vi "BRA_Query.vi"(0 "System no.":i32=1 min=1 max=4 step=1, 2 "Axes to query":string[](array[string]), 3 "Invert order?":bool, 4 "Query status of all brakes?":bool, 5 "error in":errorcluster) -> (14 "Axes with brake":string[](array[string]), 15 "Brake status?":bool[](array[boolean]), 19 "error out":errorcluster)   [LabVIEW 2020]
doc: "Returns list of axes with a brake and status of the brakes for queried axes. Requires SPA?.vi to be present.\n\nC-843, C-843.PM, C-844, Mercury: Invert order should be FALSE. Brake status? is not valid.\n\nC-848, C-880: Invert order should be TRUE. Brake status? is not valid\n\nC-884, C-891, Mercury_GCS: Invert order is not valid. VI returns axes with brakes and their brake status."
uses:
  Global1.vi
  Global2 (Array).vi
panel:
  # "Returns list of axes with a brake and status of the brakes for queried axes.  Requires \nSPA?.vi to be present."
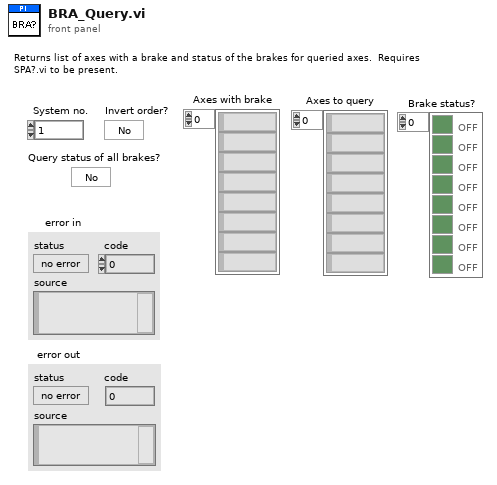
[diagram p1: front panel]
types:
  T1 = typedef "Controller names.ctl" = enum16{"None", "Analog", "C-702", "C-413", "C-414", "C-843", "C-843.PM", "C-844", "C-848", "C-865", "C-866", "C-867", "C-877", "C-880", "C-884", "C-885", "C-886", "C-887", "C-891", "E-135", "E-516", "E-517", "E-518", "E-709", "E-710", "E-712", "E-725", "E-727", "E-753", "E-754", "E-755", "E-761", "E-816", "E-861", "E-870", "E-871", "E-872", "E-873", "E-874", "F-206", "HydraPollux", "M-840", "M-850", "M-8X0", "Mercury", "Mercury_GCS", "PI_GCS2"}
  T2 = cluster{"Conn. axes":string[], "Controller name":T1}[]
  T3 = typedef "Syntax.ctl" = enum16{"GCS 1.0", "GCS 2.0", "GCS 3.0"}
  T4 = cluster{"Conn. axes":string[], "Controller name":T1}
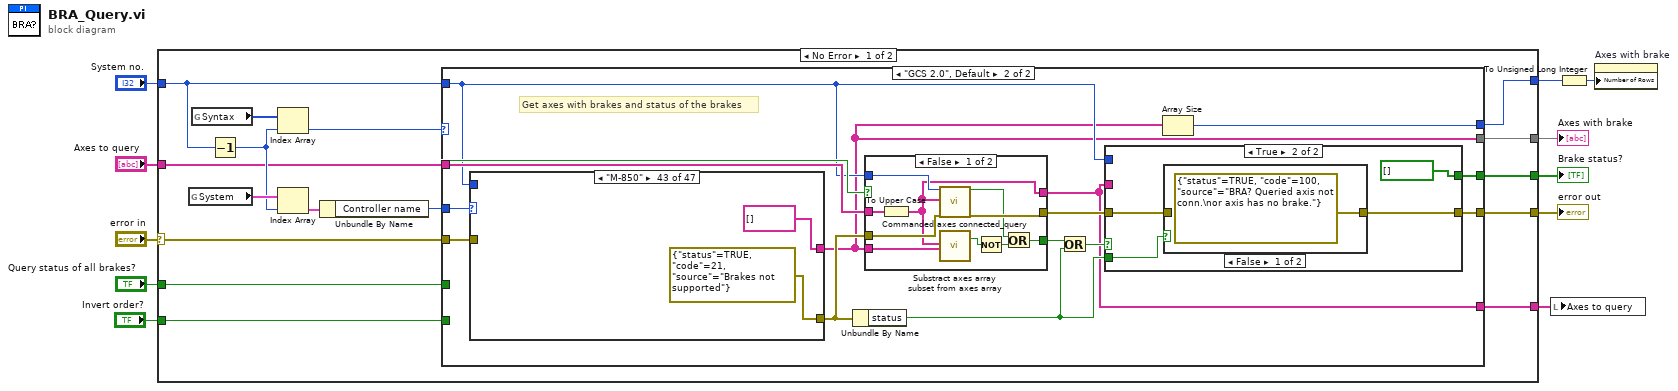
[diagram p0: block diagram]
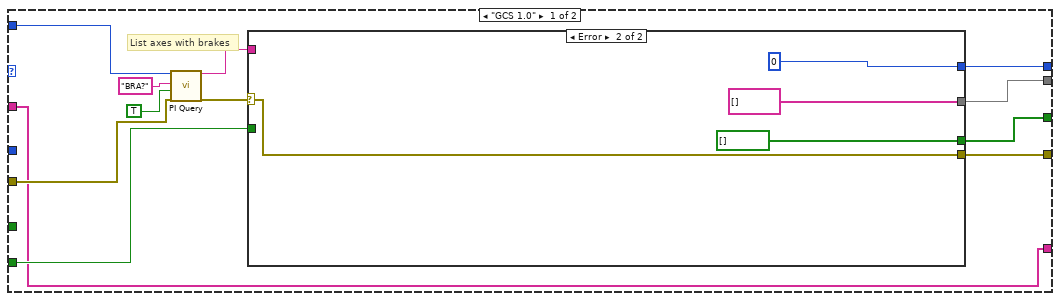
[diagram p2: hidden frame]
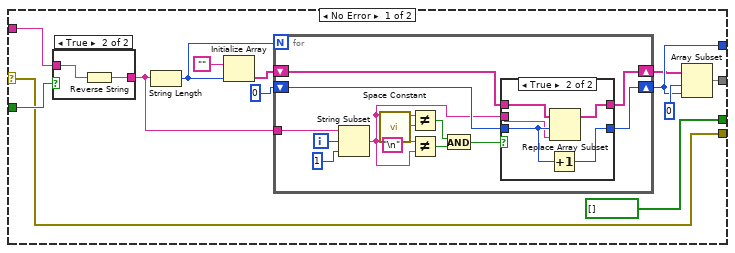
[diagram p3: hidden frame]
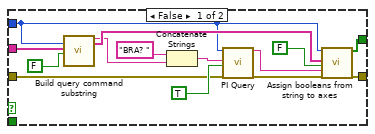
[diagram p6: hidden frame]
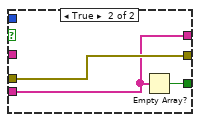
[diagram p8: hidden frame]
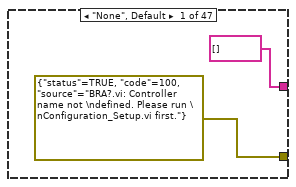
[diagram p9: hidden frame]
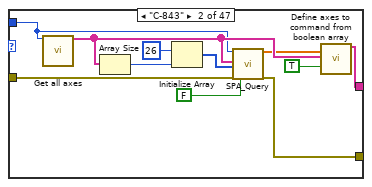
[diagram p10: hidden frame]
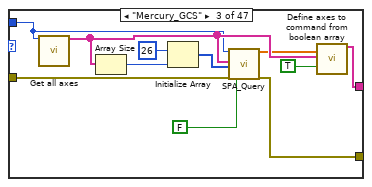
[diagram p11: hidden frame]
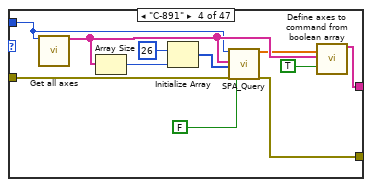
[diagram p12: hidden frame]
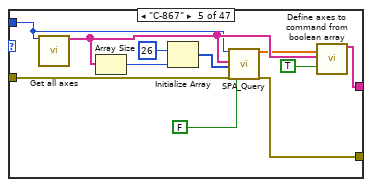
[diagram p13: hidden frame]
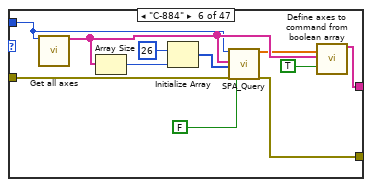
[diagram p14: hidden frame]
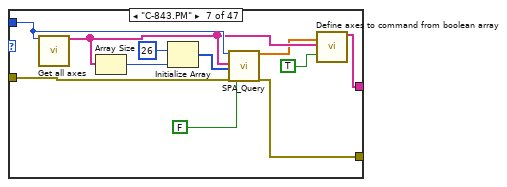
[diagram p15: hidden frame]
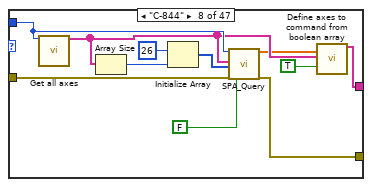
[diagram p16: hidden frame]
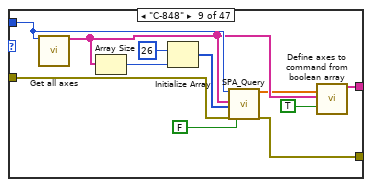
[diagram p17: hidden frame]
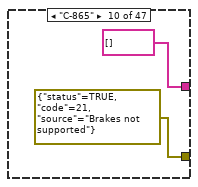
[diagram p18: hidden frame]
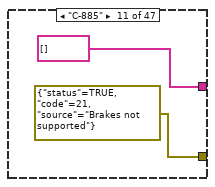
[diagram p19: hidden frame]
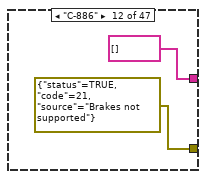
[diagram p20: hidden frame]
diagram:
  n1 = case shown="No Error" "error in" {
    selector: "error in" -> [w18 w322]
    tunnel: [w19 w322] -> w11
    tunnel: [w26 0 ("Array size out")] -> w10
    tunnel: [w25 string[] [] ("Strings")] -> w9
    tunnel: [w24 bool[] [] ("Brake status?")] -> w8
    tunnel: "System no." -> [w17 _]
    tunnel: "Query status of all brakes?" -> [w16 _]
    tunnel: "Axes to query" -> [w15 w321]
    tunnel: [w14 w321] -> w2
    tunnel: "Invert order?" -> [w12 _]
    frame No Error {
      n2 = global read "Global2 (Array).vi" "System"() -> (w23:T2)
      n3 = global read "Global1.vi" "Syntax"() -> (w27:T3[])
      n4 = Decrement(x=w17) -> (x-1=w22:i32)
      n5 = Index Array(array=w27, index=w22) -> (element=w13:T3)
      n6 = Index Array(array=w23, index=w22) -> (element=w21:T4)
      n7 = Unbundle By Name(w21) -> ("Controller name"=w20:T1)
      n8 = case shown="\"GCS 2.0\", Default" w13 {
        tunnel: [w39 w82] -> w26
        tunnel: [w38 w81] -> w25
        tunnel: w12 -> [w37 _]
        tunnel: [w36 w86] -> w24
        tunnel: w20 -> [_ w94]
        tunnel: w18 -> [w32 w93]
        tunnel: [w31 w85] -> w19
        tunnel: w16 -> [_ w92]
        tunnel: w15 -> [w28 w91]
        tunnel: w17 -> [w33 w90]
        tunnel: [w28 w80] -> w14
        frame "GCS 1.0" {
          # "List axes with brakes"
          n9 = call "PI Query.vi"("System no."=w33, "String to send"="BRA?", "Attach termination char.?"=TRUE ("Attach Linefeed?"), "error in"=w32) -> ("String read"=w30:string, "error out"=w29:errorcluster)  [unwired: 3 in, 11 out]
          n10 = case shown="Error" w29 {
            selector: w29 -> [w40 w76]
            tunnel: [w47 0] -> w39
            tunnel: [w45 string[] []] -> w38
            tunnel: w30 -> [w44 _]
            tunnel: w37 -> [w42 _]
            tunnel: [bool[] [] ("Brake status?") bool[] [] ("Brake status?")] -> w36
            tunnel: [w40 w76] -> w31
            frame No Error {
              n11 = case shown="True" w42 {
                tunnel: w44 -> [w53 w55]
                tunnel: [w53 w54] -> w43
                frame False {
                }
                frame True {
                  n12 = Reverse String(1:w55) -> (0:w54:string)
                }
              }
              n13 = String Length(string=w43) -> (length=w51:i32)
              n14 = Initialize Array("" ("Element Data"), w51) -> (w49:string[])
              n15 = for {
                N: w51 -> [_]
                tunnel: w43 -> [w68]
                shift-right: [w61] -> w46
                shift-left: w49 -> [w62]
                shift-right: [w64] -> w47
                shift-left: 0 -> [w63]
                i -> [w66]
                n16 = String Subset(string=w68, offset (0)=w66, length (rest)=1 ("length")) -> (substring=w60:string)
                n17 = call "Space Constant.vi"() -> ("String"=w65:string)
                n18 = Not Equal?(x=w60, y=w65) -> (x != y?=w58:bool)
                n19 = Not Equal?(x="\n", y=w60) -> (x != y?=w57:bool)
                n20 = And(x=w58, y=w57) -> (x .and. y?=w56:bool)
                n21 = case shown="True" w56 {
                  tunnel: [w70 w75] -> w64
                  tunnel: w63 -> [w70 w73]
                  tunnel: w62 -> [w69 w74]
                  tunnel: w60 -> [_ w72]
                  tunnel: [w69 w71] -> w61
                  frame False {
                  }
                  frame True {
                    n22 = Increment(x=w73) -> (x+1=w75:i32)
                    n23 = Replace Array Subset(array=w74, new element=w72, index=w73) -> (w71:string[])
                  }
                }
              }
              n24 = Array Subset(array=w46, index=0 ("Array Index"), length=w47) -> (w45:string[])
            }
            frame Error {
            }
          }
        }
        frame "GCS 2.0", Default {
          # "Get axes with brakes and status of the brakes"
          n25 = case shown="\"M-850\"" w94 {
            tunnel: w90 -> [_ w130 w141 w152 w163 w174 w195 w206 w217 _ _ _ _ _ _ _ _ _ _ _ _ _ _ _ _ _ _ _ _ _ _ _ _ _ _ _ _ _ _ _ _ _ _ _ w298 w309 w320]
            tunnel: w93 -> [_ w137 w148 w159 w170 w181 w191 w202 w213 _ _ _ _ _ _ _ _ _ _ _ _ _ _ _ _ _ _ _ _ _ _ _ _ _ _ _ _ _ _ _ _ _ _ _ w294 w305 w316]
            tunnel: [errorcluster {"status"=TRUE, "code"=100, "source"="BRA?.vi: Controller name not \ndefined. Please run \nConfiguration_Setup.vi first."} ("error out") w135 w146 w157 w168 w179 w189 w200 w211 errorcluster {"status"=TRUE, "code"=21, "source"="Brakes not supported"} ("error out") errorcluster {"status"=TRUE, "code"=21, "source"="Brakes not supported"} ("error out") errorcluster {"status"=TRUE, "code"=21, "source"="Brakes not supported"} ("error out") errorcluster {"status"=TRUE, "code"=21, "source"="Brakes not supported"} ("error out") errorcluster {"status"=TRUE, "code"=21, "source"="Brakes not supported"} ("error out") errorcluster {"status"=TRUE, "code"=21, "source"="Brakes not supported"} ("error out") errorcluster {"status"=TRUE, "code"=21, "source"="Brakes not supported"} ("error out") errorcluster {"status"=TRUE, "code"=21, "source"="Brakes not supported"} ("error out") errorcluster {"status"=TRUE, "code"=21, "source"="Brakes not supported"} ("error out") errorcluster {"status"=TRUE, "code"=21, "source"="Brakes not supported"} ("error out") errorcluster {"status"=TRUE, "code"=21, "source"="Brakes not supported"} ("error out") errorcluster {"status"=TRUE, "code"=21, "source"="Brakes not supported"} ("error out") errorcluster {"status"=TRUE, "code"=21, "source"="Brakes not supported"} ("error out") errorcluster {"status"=TRUE, "code"=21, "source"="Brakes not supported"} ("error out") errorcluster {"status"=TRUE, "code"=21, "source"="Brakes not supported"} ("error out") errorcluster {"status"=TRUE, "code"=21, "source"="Brakes not supported"} ("error out") errorcluster {"status"=TRUE, "code"=21, "source"="Brakes not supported"} ("error out") errorcluster {"status"=TRUE, "code"=21, "source"="Brakes not supported"} ("error out") errorcluster {"status"=TRUE, "code"=21, "source"="Brakes not supported"} ("error out") errorcluster {"status"=TRUE, "code"=21, "source"="Brakes not supported"} ("error out") errorcluster {"status"=TRUE, "code"=21, "source"="Brakes not supported"} ("error out") errorcluster {"status"=TRUE, "code"=21, "source"="Brakes not supported"} ("error out") errorcluster {"status"=TRUE, "code"=21, "source"="Brakes not supported"} ("error out") errorcluster {"status"=TRUE, "code"=21, "source"="Brakes not supported"} ("error out") errorcluster {"status"=TRUE, "code"=21, "source"="Brakes not supported"} ("error out") errorcluster {"status"=TRUE, "code"=21, "source"="Brakes not supported"} ("error out") errorcluster {"status"=TRUE, "code"=21, "source"="Brakes not supported"} ("error out") errorcluster {"status"=TRUE, "code"=21, "source"="Brakes not supported"} ("error out") errorcluster {"status"=TRUE, "code"=21, "source"="Brakes not supported"} ("error out") errorcluster {"status"=TRUE, "code"=21, "source"="Brakes not supported"} ("error out") errorcluster {"status"=TRUE, "code"=21, "source"="Brakes not supported"} ("error out") errorcluster {"status"=TRUE, "code"=21, "source"="Brakes not supported"} ("error out") errorcluster {"status"=TRUE, "code"=21, "source"="Brakes not supported"} ("error out") errorcluster {"status"=TRUE, "code"=21, "source"="Brakes not supported"} ("error out") errorcluster {"status"=TRUE, "code"=21, "source"="Brakes not supported"} ("error out") w292 w303 w314] -> w83
            tunnel: [string[] [] ("Axes to command") w132 w143 w154 w165 w176 w186 w197 w208 string[] [] ("Axes to command") string[] [] ("Axes to command") string[] [] ("Axes to command") string[] [] ("Axes to command") string[] [] ("Axes to command") string[] [] ("Axes to command") string[] [] ("Axes to command") string[] [] ("Axes to command") string[] [] ("Axes to command") string[] [] ("Axes to command") string[] [] ("Axes to command") string[] [] ("Axes to command") string[] [] ("Axes to command") string[] [] ("Axes to command") string[] [] ("Axes to command") string[] [] ("Axes to command") string[] [] ("Axes to command") string[] [] ("Axes to command") string[] [] ("Axes to command") string[] [] ("Axes to command") string[] [] ("Axes to command") string[] [] ("Axes to command") string[] [] ("Axes to command") string[] [] ("Axes to command") string[] [] ("Axes to command") string[] [] ("Axes to command") string[] [] ("Axes to command") string[] [] ("Axes to command") string[] [] ("Axes to command") string[] [] ("Axes to command") string[] [] ("Axes to command") string[] [] ("Axes to command") string[] [] ("Axes to command") string[] [] ("Axes to command") string[] [] ("Axes to command") w289 w300 w311] -> w81
            frame "None", Default {
            }
            frame "C-843" {
              n26 = call "Get all axes.vi"("System no."=w130) -> ("Conn. Axes"=w134:string[])  [unwired: 18 out]
              n27 = Array Size(array=w134) -> (size(s)=w140:i32)
              n28 = Initialize Array(26, w140) -> (w138:i32[])
              n29 = call "SPA_Query.vi"("System no."=w130, "Axes to query"=w134, "Parameter no."=w138, "error in"=w137, "Parameter no. format \n(Decimal: FALSE)"=FALSE ("Parameter no. format \n(Decimal: FALSE)")) -> ("Parameter value"=w131:dbl[], "error out"=w135:errorcluster)  [unwired: 2 in, 11 out]
              n30 = call "Define axes to command from boolean array.vi"("Command axis? (num)"=w131, "Axes to query"=w134, "Command axis? format\n(Boolean: FALSE)"=TRUE ("Command axis? format\n(Boolean: FALSE)")) -> ("Axes to command"=w132:string[])  [unwired: 2 in, 14 out]
            }
            frame "Mercury_GCS" {
              n31 = call "Get all axes.vi"("System no."=w141) -> ("Conn. Axes"=w145:string[])  [unwired: 18 out]
              n32 = Array Size(array=w145) -> (size(s)=w151:i32)
              n33 = Initialize Array(26, w151) -> (w149:i32[])
              n34 = call "SPA_Query.vi"("System no."=w141, "Axes to query"=w145, "Parameter no."=w149, "error in"=w148, "Parameter no. format \n(Decimal: FALSE)"=FALSE ("Parameter no. format \n(Decimal: FALSE)")) -> ("Parameter value"=w142:dbl[], "error out"=w146:errorcluster)  [unwired: 2 in, 11 out]
              n35 = call "Define axes to command from boolean array.vi"("Command axis? (num)"=w142, "Axes to query"=w145, "Command axis? format\n(Boolean: FALSE)"=TRUE ("Command axis? format\n(Boolean: FALSE)")) -> ("Axes to command"=w143:string[])  [unwired: 2 in, 14 out]
            }
            frame "C-891" {
              n36 = call "Get all axes.vi"("System no."=w152) -> ("Conn. Axes"=w156:string[])  [unwired: 18 out]
              n37 = Array Size(array=w156) -> (size(s)=w162:i32)
              n38 = Initialize Array(26, w162) -> (w160:i32[])
              n39 = call "SPA_Query.vi"("System no."=w152, "Axes to query"=w156, "Parameter no."=w160, "error in"=w159, "Parameter no. format \n(Decimal: FALSE)"=FALSE ("Parameter no. format \n(Decimal: FALSE)")) -> ("Parameter value"=w153:dbl[], "error out"=w157:errorcluster)  [unwired: 2 in, 11 out]
              n40 = call "Define axes to command from boolean array.vi"("Command axis? (num)"=w153, "Axes to query"=w156, "Command axis? format\n(Boolean: FALSE)"=TRUE ("Command axis? format\n(Boolean: FALSE)")) -> ("Axes to command"=w154:string[])  [unwired: 2 in, 14 out]
            }
            frame "C-867" {
              n41 = call "Get all axes.vi"("System no."=w163) -> ("Conn. Axes"=w167:string[])  [unwired: 18 out]
              n42 = Array Size(array=w167) -> (size(s)=w173:i32)
              n43 = Initialize Array(26, w173) -> (w171:i32[])
              n44 = call "SPA_Query.vi"("System no."=w163, "Axes to query"=w167, "Parameter no."=w171, "error in"=w170, "Parameter no. format \n(Decimal: FALSE)"=FALSE ("Parameter no. format \n(Decimal: FALSE)")) -> ("Parameter value"=w164:dbl[], "error out"=w168:errorcluster)  [unwired: 2 in, 11 out]
              n45 = call "Define axes to command from boolean array.vi"("Command axis? (num)"=w164, "Axes to query"=w167, "Command axis? format\n(Boolean: FALSE)"=TRUE ("Command axis? format\n(Boolean: FALSE)")) -> ("Axes to command"=w165:string[])  [unwired: 2 in, 14 out]
            }
            frame "C-884" {
              n46 = call "Get all axes.vi"("System no."=w174) -> ("Conn. Axes"=w178:string[])  [unwired: 18 out]
              n47 = Array Size(array=w178) -> (size(s)=w184:i32)
              n48 = Initialize Array(26, w184) -> (w182:i32[])
              n49 = call "SPA_Query.vi"("System no."=w174, "Axes to query"=w178, "Parameter no."=w182, "error in"=w181, "Parameter no. format \n(Decimal: FALSE)"=FALSE ("Parameter no. format \n(Decimal: FALSE)")) -> ("Parameter value"=w175:dbl[], "error out"=w179:errorcluster)  [unwired: 2 in, 11 out]
              n50 = call "Define axes to command from boolean array.vi"("Command axis? (num)"=w175, "Axes to query"=w178, "Command axis? format\n(Boolean: FALSE)"=TRUE ("Command axis? format\n(Boolean: FALSE)")) -> ("Axes to command"=w176:string[])  [unwired: 2 in, 14 out]
            }
            frame "C-843.PM" {
              n51 = call "Get all axes.vi"("System no."=w195) -> ("Conn. Axes"=w188:string[])  [unwired: 18 out]
              n52 = Array Size(array=w188) -> (size(s)=w194:i32)
              n53 = Initialize Array(26, w194) -> (w192:i32[])
              n54 = call "SPA_Query.vi"("System no."=w195, "Axes to query"=w188, "Parameter no."=w192, "error in"=w191, "Parameter no. format \n(Decimal: FALSE)"=FALSE ("Parameter no. format \n(Decimal: FALSE)")) -> ("Parameter value"=w185:dbl[], "error out"=w189:errorcluster)  [unwired: 2 in, 11 out]
              n55 = call "Define axes to command from boolean array.vi"("Command axis? (num)"=w185, "Axes to query"=w188, "Command axis? format\n(Boolean: FALSE)"=TRUE ("Command axis? format\n(Boolean: FALSE)")) -> ("Axes to command"=w186:string[])  [unwired: 2 in, 14 out]
            }
            frame "C-844" {
              n56 = call "Get all axes.vi"("System no."=w206) -> ("Conn. Axes"=w199:string[])  [unwired: 18 out]
              n57 = Array Size(array=w199) -> (size(s)=w205:i32)
              n58 = Initialize Array(26, w205) -> (w203:i32[])
              n59 = call "SPA_Query.vi"("System no."=w206, "Axes to query"=w199, "Parameter no."=w203, "error in"=w202, "Parameter no. format \n(Decimal: FALSE)"=FALSE ("Parameter no. format \n(Decimal: FALSE)")) -> ("Parameter value"=w196:dbl[], "error out"=w200:errorcluster)  [unwired: 2 in, 11 out]
              n60 = call "Define axes to command from boolean array.vi"("Command axis? (num)"=w196, "Axes to query"=w199, "Command axis? format\n(Boolean: FALSE)"=TRUE ("Command axis? format\n(Boolean: FALSE)")) -> ("Axes to command"=w197:string[])  [unwired: 2 in, 14 out]
            }
            frame "C-848" {
              n61 = call "Get all axes.vi"("System no."=w217) -> ("Conn. Axes"=w210:string[])  [unwired: 18 out]
              n62 = Array Size(array=w210) -> (size(s)=w216:i32)
              n63 = Initialize Array(26, w216) -> (w214:i32[])
              n64 = call "SPA_Query.vi"("System no."=w217, "Axes to query"=w210, "Parameter no."=w214, "error in"=w213, "Parameter no. format \n(Decimal: FALSE)"=FALSE ("Parameter no. format \n(Decimal: FALSE)")) -> ("Parameter value"=w207:dbl[], "error out"=w211:errorcluster)  [unwired: 2 in, 11 out]
              n65 = call "Define axes to command from boolean array.vi"("Command axis? (num)"=w207, "Axes to query"=w210, "Command axis? format\n(Boolean: FALSE)"=TRUE ("Command axis? format\n(Boolean: FALSE)")) -> ("Axes to command"=w208:string[])  [unwired: 2 in, 14 out]
            }
            frame "C-865" {
            }
            frame "C-885" {
            }
            frame "C-886" {
            }
            frame "C-887" {
            }
            frame "E-870" {
            }
            frame "E-871" {
            }
            frame "E-872" {
            }
            frame "HydraPollux" {
            }
            frame "C-413" {
            }
            frame "C-414" {
            }
            frame "E-135" {
            }
            frame "C-877" {
            }
            frame "E-518" {
            }
            frame "E-727" {
            }
            frame "E-754" {
            }
            frame "E-873" {
            }
            frame "E-874" {
            }
            frame "E-709" {
            }
            frame "C-866" {
            }
            frame "E-517" {
            }
            frame "E-712" {
            }
            frame "E-725" {
            }
            frame "E-753" {
            }
            frame "E-755" {
            }
            frame "E-861" {
            }
            frame "Analog" {
            }
            frame "C-702" {
            }
            frame "E-516" {
            }
            frame "E-710" {
            }
            frame "E-761" {
            }
            frame "E-816" {
            }
            frame "F-206" {
            }
            frame "M-840" {
            }
            frame "M-850" {
            }
            frame "M-8X0" {
            }
            frame "C-880" {
              n66 = call "Get all axes.vi"("System no."=w298) -> ("Conn. Axes"=w291:string[])  [unwired: 18 out]
              n67 = Array Size(array=w291) -> (size(s)=w297:i32)
              n68 = Initialize Array(26, w297) -> (w295:i32[])
              n69 = call "SPA_Query.vi"("System no."=w298, "Axes to query"=w291, "Parameter no."=w295, "error in"=w294, "Parameter no. format \n(Decimal: FALSE)"=FALSE ("Parameter no. format \n(Decimal: FALSE)")) -> ("Parameter value"=w288:dbl[], "error out"=w292:errorcluster)  [unwired: 2 in, 11 out]
              n70 = call "Define axes to command from boolean array.vi"("Command axis? (num)"=w288, "Axes to query"=w291, "Command axis? format\n(Boolean: FALSE)"=TRUE ("Command axis? format\n(Boolean: FALSE)")) -> ("Axes to command"=w289:string[])  [unwired: 2 in, 14 out]
            }
            frame "Mercury" {
              n71 = call "Get all axes.vi"("System no."=w309) -> ("Conn. Axes"=w302:string[])  [unwired: 18 out]
              n72 = Array Size(array=w302) -> (size(s)=w308:i32)
              n73 = Initialize Array(26, w308) -> (w306:i32[])
              n74 = call "SPA_Query.vi"("System no."=w309, "Axes to query"=w302, "Parameter no."=w306, "error in"=w305, "Parameter no. format \n(Decimal: FALSE)"=FALSE ("Parameter no. format \n(Decimal: FALSE)")) -> ("Parameter value"=w299:dbl[], "error out"=w303:errorcluster)  [unwired: 2 in, 11 out]
              n75 = call "Define axes to command from boolean array.vi"("Command axis? (num)"=w299, "Axes to query"=w302, "Command axis? format\n(Boolean: FALSE)"=TRUE ("Command axis? format\n(Boolean: FALSE)")) -> ("Axes to command"=w300:string[])  [unwired: 2 in, 14 out]
            }
            frame "PI_GCS2" {
              n76 = call "Get all axes.vi"("System no."=w320) -> ("Conn. Axes"=w313:string[])  [unwired: 18 out]
              n77 = Array Size(array=w313) -> (size(s)=w319:i32)
              n78 = Initialize Array(26, w319) -> (w317:i32[])
              n79 = call "SPA_Query.vi"("System no."=w320, "Axes to query"=w313, "Parameter no."=w317, "error in"=w316, "Parameter no. format \n(Decimal: FALSE)"=FALSE ("Parameter no. format \n(Decimal: FALSE)")) -> ("Parameter value"=w310:dbl[], "error out"=w314:errorcluster)  [unwired: 2 in, 11 out]
              n80 = call "Define axes to command from boolean array.vi"("Command axis? (num)"=w310, "Axes to query"=w313, "Command axis? format\n(Boolean: FALSE)"=TRUE ("Command axis? format\n(Boolean: FALSE)")) -> ("Axes to command"=w311:string[])  [unwired: 2 in, 14 out]
            }
          }
          n81 = Unbundle By Name(w83) -> ("status"=w84:bool)
          n82 = case shown="False" w92 {
            tunnel: [w119 w126] -> w80
            tunnel: w81 -> [w120 w126]
            tunnel: w91 -> [w124 _]
            tunnel: w90 -> [w123 _]
            tunnel: w83 -> [w122 w127]
            tunnel: [w121 w127] -> w88
            tunnel: [w115 w125] -> w89
            frame False {
              n83 = To Upper Case(1:w124) -> (0:w119:string[])
              n84 = call "Commanded axes connected_query.vi"("System no."=w123, "Commanded axes"=w119, "error in"=w122) -> ("Controller error"=w117:bool, "error out"=w121:errorcluster)  [unwired: 1 in, 14 out]
              n85 = call "Substract axes array subset from axes array.vi"("Axes to query"=w119, "Axes subset"=w120) -> ("All present?"=w118:bool)  [unwired: 17 out]
              n86 = Not(x=w118) -> (.not. x?=w116:bool)
              n87 = Or(x=w117, y=w116) -> (x .or. y?=w115:bool)
            }
            frame True {
              n88 = Empty Array?(array=w126) -> (empty?=w125:bool)
            }
          }
          n89 = Or(x=w89, y=w84) -> (x .or. y?=w87:bool)
          n90 = case shown="True" w87 {
            tunnel: w88 -> [w103 w109]
            tunnel: w80 -> [w101 _]
            tunnel: w90 -> [w100 _]
            tunnel: [w99 bool[] [] ("Booleans")] -> w86
            tunnel: [w98 w110] -> w85
            tunnel: w84 -> [_ w111]
            frame False {
              n91 = call "Build query command substring.vi"("System no."=w100, "Axes to query in"=w101, "Query\nAll axes?"=FALSE ("Query\nAll axes?")) -> ("Command substring"=w107:string, "Axes to query out"=w108:string[])  [unwired: 3 in, 12 out]
              n92 = Concatenate Strings("BRA? ", w107) -> (w106:string)
              n93 = call "PI Query.vi"("System no."=w100, "String to send"=w106, "Attach termination char.?"=TRUE ("Attach Linefeed?"), "error in"=w103) -> ("String read"=w96:string, "error out"=w95:errorcluster)  [unwired: 3 in, 11 out]
              n94 = call "Assign booleans from string to axes.vi"("System no."=w100, "Queried axes"=w108, "All axes queried?"=FALSE, "Input String"=w96, "error in"=w95) -> ("Booleans"=w99:bool[], "error out"=w98:errorcluster)  [unwired: 13 out]
            }
            frame True {
              n95 = case shown="False" w111 {
                tunnel: w109 -> [_ w114]
                tunnel: [errorcluster {"status"=TRUE, "code"=100, "source"="BRA? Queried axis not conn.\nor axis has no brake."} ("error out") w114] -> w110
                frame False {
                }
                frame True {
                }
              }
            }
          }
          n96 = Array Size(array=w81) -> (size(s)=w82:i32)
        }
      }
    }
    frame Error {
    }
  }
  "Axes with brake" <- w9
  "error out" <- w11
  "Brake status?" <- w8
  n97 = local write "Axes to query"(w2) -> ()
  n98 = To Unsigned Long Integer(number=w10) -> (unsigned 32bit integer=w7:u32)
  n99 = property on="Axes with brake" class="Arr (strict)"("Number of Rows"=w7) -> ()  [unwired: 2 in, 2 out]
